vi "READTEMP.vi"(2 "Lakeshore Address":string="13", 3 "Wait Time (s)":sgl=10.0 min=10 max=1e+09 format="%<%H:%M:%S%0u>t", 4 "units":i8(ring) items=["K", "C", "F", "ohms"], 6 "?":bool) -> (0 "cycles":i32, 1 "?":dbl(graph), 5 "Temperature output":ext format="%.2f")   [LabVIEW 2020]
panel:
  in  "limit cycle":i32
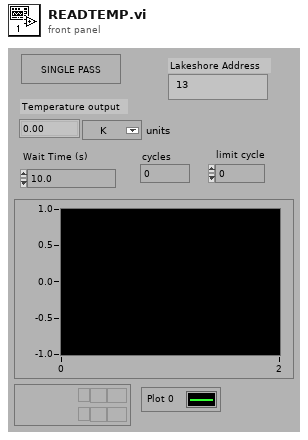
[diagram p1: front panel]
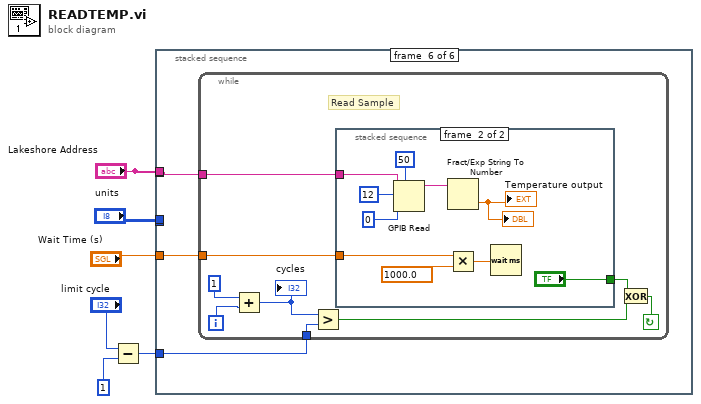
[diagram p0: block diagram]
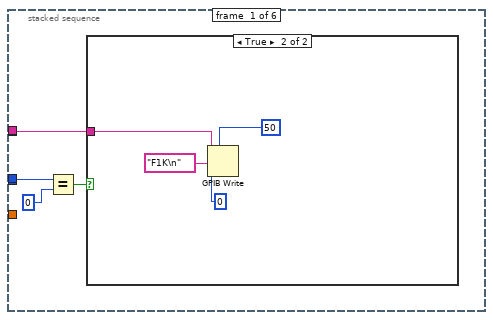
[diagram p2: hidden frame]
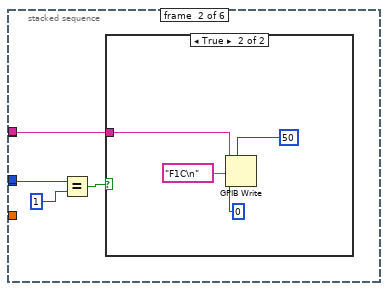
[diagram p4: hidden frame]
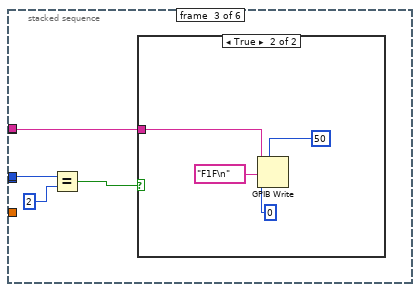
[diagram p6: hidden frame]
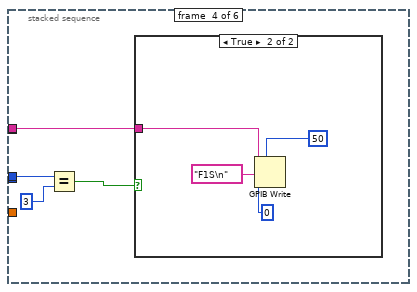
[diagram p8: hidden frame]
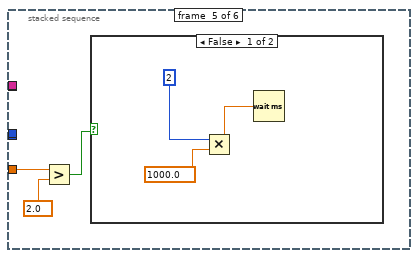
[diagram p10: hidden frame]
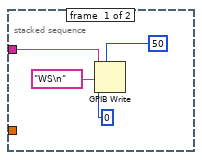
[diagram p12: hidden frame]
diagram:
  n1 = Subtract(x="limit cycle", y=1) -> (x-y=w1:i32)
  n2 = stacked-sequence {
    tunnel: "units" -> [w10 _ _ _ _ _]
    tunnel: "units" -> [_ w15 _ _ _ _]
    tunnel: "units" -> [_ _ w23 w32 _ _]
    tunnel: "Lakeshore Address" -> [w7 w16 w24 _ _ w47]
    tunnel: "Lakeshore Address" -> [_ _ _ w31 _ _]
    tunnel: "Wait Time (s)" -> [_ _ _ _ w40 w46]
    tunnel: w1 -> [_ _ _ _ _ w45]
    frame #0 {
      n3 = Equal?(x=w10, y=0) -> (x = y?=w8:bool)
      n4 = case shown="True" w8 {
        tunnel: w7 -> [_ w11]
        frame False {
        }
        frame True {
          n5 = GPIB Write(0:w11, 1:"F1K\n", 2:0, 4:50) -> ()  [unwired: 1 in, 2 out]
        }
      }
    }
    frame #1 {
      n6 = Equal?(x=w15, y=1) -> (x = y?=w17:bool)
      n7 = case shown="True" w17 {
        tunnel: w16 -> [_ w19]
        frame False {
        }
        frame True {
          n8 = GPIB Write(0:w19, 1:"F1C\n", 2:0, 4:50) -> ()  [unwired: 1 in, 2 out]
        }
      }
    }
    frame #2 {
      n9 = Equal?(x=w23, y=2) -> (x = y?=w25:bool)
      n10 = case shown="True" w25 {
        tunnel: w24 -> [_ w27]
        frame False {
        }
        frame True {
          n11 = GPIB Write(0:w27, 1:"F1F\n", 2:0, 4:50) -> ()  [unwired: 1 in, 2 out]
        }
      }
    }
    frame #3 {
      n12 = Equal?(x=w32, y=3) -> (x = y?=w33:bool)
      n13 = case shown="True" w33 {
        tunnel: w31 -> [_ w35]
        frame False {
        }
        frame True {
          n14 = GPIB Write(0:w35, 1:"F1S\n", 2:0, 4:50) -> ()  [unwired: 1 in, 2 out]
        }
      }
    }
    frame #4 {
      n15 = Greater?(x=w40, y=2.0) -> (0:w41:bool)
      n16 = case shown="False" w41 {
        frame False {
          n17 = Multiply(x=2, y=1000.0) -> (x*y=w43:dbl)
          n18 = Wait (ms)(milliseconds to wait=w43) -> ()  [unwired: 1 out]
        }
        frame True {
        }
      }
    }
    frame #5 {
      n19 = while {
        tunnel: w45 -> [w51]
        tunnel: w46 -> [w53]
        tunnel: w47 -> [w56]
        i -> [w54]
        stop <- w48 continue-if-true
        (unwired) 170.89
        # "Read Sample"
        n20 = Add(x=1, y=w54) -> (x+y=w52:i32)
        "cycles" <- w52
        n21 = Greater?(x=w52, y=w51) -> (0:w49:bool)
        n22 = stacked-sequence {
          tunnel: w56 -> [w57 w67]
          tunnel: [_ "?"] -> w50
          tunnel: w53 -> [_ w61]
          frame #0 {
            n23 = GPIB Write(0:w57, 1:"WS\n", 2:0, 4:50) -> ()  [unwired: 1 in, 2 out]
          }
          frame #1 {
            n24 = GPIB Read(0:w67, 1:12, 2:0, 4:50) -> (5:w68:string)  [unwired: 1 in, 2 out]
            n25 = Fract/Exp String To Number(string=w68) -> (number=→"Temperature output" →"?":dbl)  [unwired: 3 in, 1 out]
            n26 = Multiply(x=w61, y=1000.0) -> (x*y=w63:dbl)
            n27 = Wait (ms)(milliseconds to wait=w63) -> ()  [unwired: 1 out]
          }
        }
        n28 = Exclusive Or(1:w49, 2:w50) -> (0:w48:bool)
      }
    }
  }
